vi "Get_Keys.vi"(0 "Target_Data":map{string, refnum<class "I2C.lvclass">}(c390)) -> (4 "Keys_and_Index":cluster{"String":string, "Value":u16}[](array[cluster]), 6 "Keys":string[](array[string]), 8 "Elements":refnum<class "I2C.lvclass">[](array[class]), 10 "First_Key":string, 15 "First_Element":refnum<class "I2C.lvclass">)   [LabVIEW 2021]
doc: "Used to get the keys of the map"
uses:
  Class/I2C/I2C.lvclass
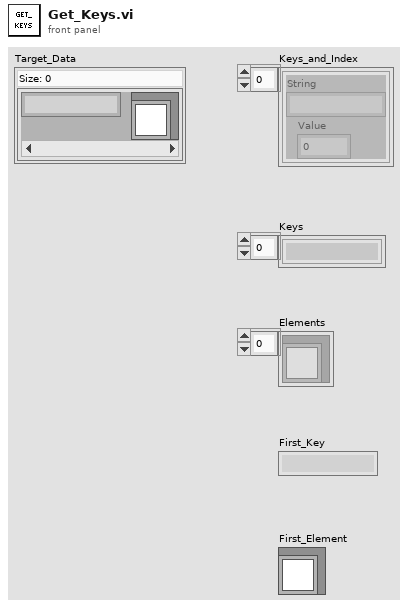
[diagram p1: front panel]
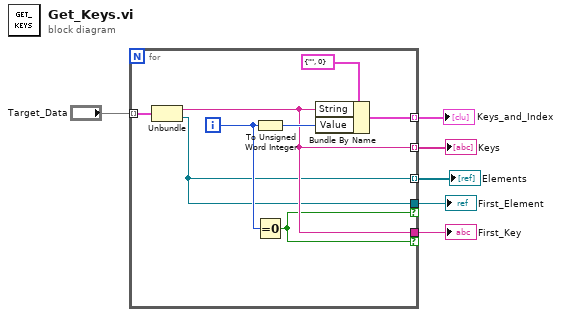
[diagram p0: block diagram]
diagram:
  n1 = for {
    tunnel: [w13] -> w6 mode=indexing
    tunnel: "Target_Data" -> [w12] mode=indexing
    tunnel: [w10] -> w4 mode=indexing
    tunnel: [w10] -> w2 if=w8
    tunnel: [w7] -> w3 if=w8
    tunnel: [w7] -> w1 mode=indexing
    i -> [w9]
    n2 = Unbundle(w12) -> (w10:string, w7:refnum<class "I2C.lvclass">)
    n3 = To Unsigned Word Integer(number=w9) -> (unsigned 16bit integer=w11:u16)
    n4 = Equal To 0?(x=w9) -> (x = 0?=w8:bool)
    n5 = Bundle By Name(cluster=cluster{"String":string, "Value":u16} {"String"="", "Value"=0} ("Cluster"), "String"=w10, "Value"=w11) -> (w13:cluster{"String":string, "Value":u16})
  }
  "Keys_and_Index" <- w6
  "Keys" <- w4
  "First_Element" <- w3
  "First_Key" <- w2
  "Elements" <- w1
